vi "Test2_3a_ruben.vi"(7 "Report Enable":bool=TRUE, 8 "error in":errorcluster, 9 "Cycles Burst":i32=10000, 11 "Instrument VISA in":T1={"AWG VISA"="81160A", "Oscilloscope  VISA "="DSO80204B", "Integration Board IP"="172.16.7.43", "connection ID"=refnum, "report out"=refnum, "report file path"=path "D:/CTA/LevelTriggerBoardTest/TestsData/sumtrigger_delay/dataruben"}) -> (0 "error out":errorcluster, 3 "Instrument VISA out":T1={"AWG VISA"="81160A", "Oscilloscope  VISA "="DSO80204B", "Integration Board IP"="172.16.7.43", "connection ID"=refnum, "report out"=refnum, "report file path"=path "D:/CTA/LevelTriggerBoardTest/TestsData/sumtrigger_delay/dataruben"})   [LabVIEW 2009]
uses:
  <vilib>/Utility/NIReport.llb/NI_report.lvclass
  <vilib>/Utility/NIReport.llb/HTML/NI_HTML.lvclass
  <instrlib>/Agilent 8000 Series/Public/Configure/Configure Math (Binary Operation).vi
  <instrlib>/Agilent 81150/Agilent 81150.lvlib
  <instrlib>/Agilent 8000 Series/Agilent 8000 Series.lvlib
panel:
  in  "Quantity of measurements":u32
  in  "Delay Time (s)":dbl=10.0
  in  "Channel":i32=1
  in  "Points":i32=360
  in  "Save NOW!":bool
  in  "End 2":bool=TRUE
  out "Data output":dbl[][](array[numeric])=[[1.0, 1.0, 2200.0, 200.0, 0.0, 0.26, nan, 1.00955e-08, nan, 2.8861e-09, nan, 0.961, nan], [1.0, 1.0, 2200.0, 200.0, 1.0, 0.261, nan, 1.0146e-08, nan, 2.9059e-09, nan, 0.961, nan]]
  in  "sweep Vclip":T2={"MIN"=200.0, "MAX"=200.0, "Steps"=1.0, "Log scale"=FALSE}
  in  "sweep Vatt":T2={"MIN"=2200.0, "MAX"=2200.0, "Steps"=1.0, "Log scale"=FALSE}
  out "Measurement":dbl=0.261
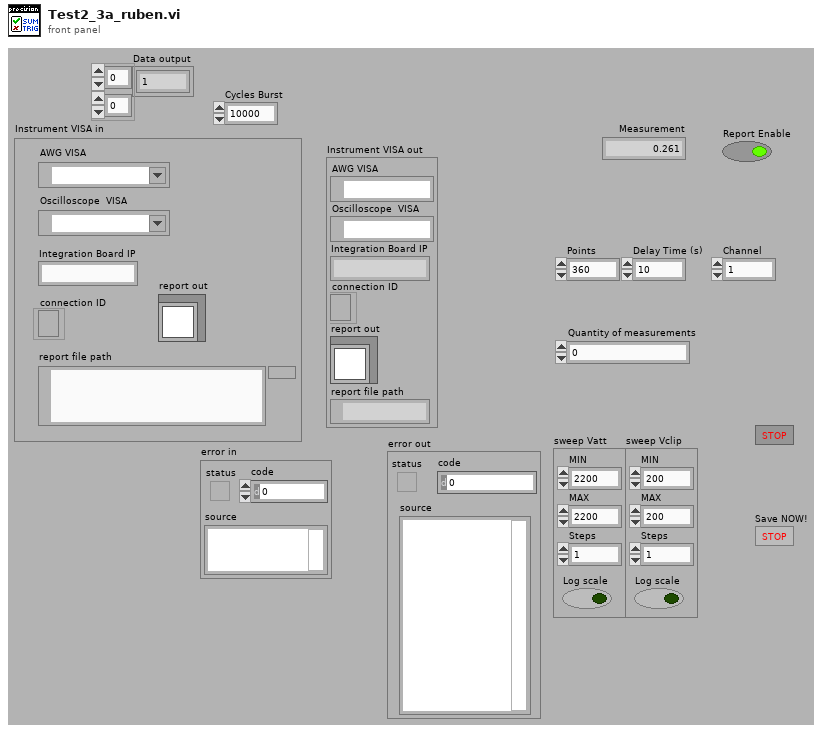
[diagram p1: front panel]
types:
  T1 = cluster{"AWG VISA":refnum<visa-resource-name>, "Oscilloscope  VISA ":refnum<visa-resource-name>, "Integration Board IP":string, "connection ID":refnum<k5>, "report out":refnum<class "NI_report.lvclass">, "report file path":path}
  T2 = cluster{"MIN":dbl, "MAX":dbl, "Steps":dbl, "Log scale":bool}
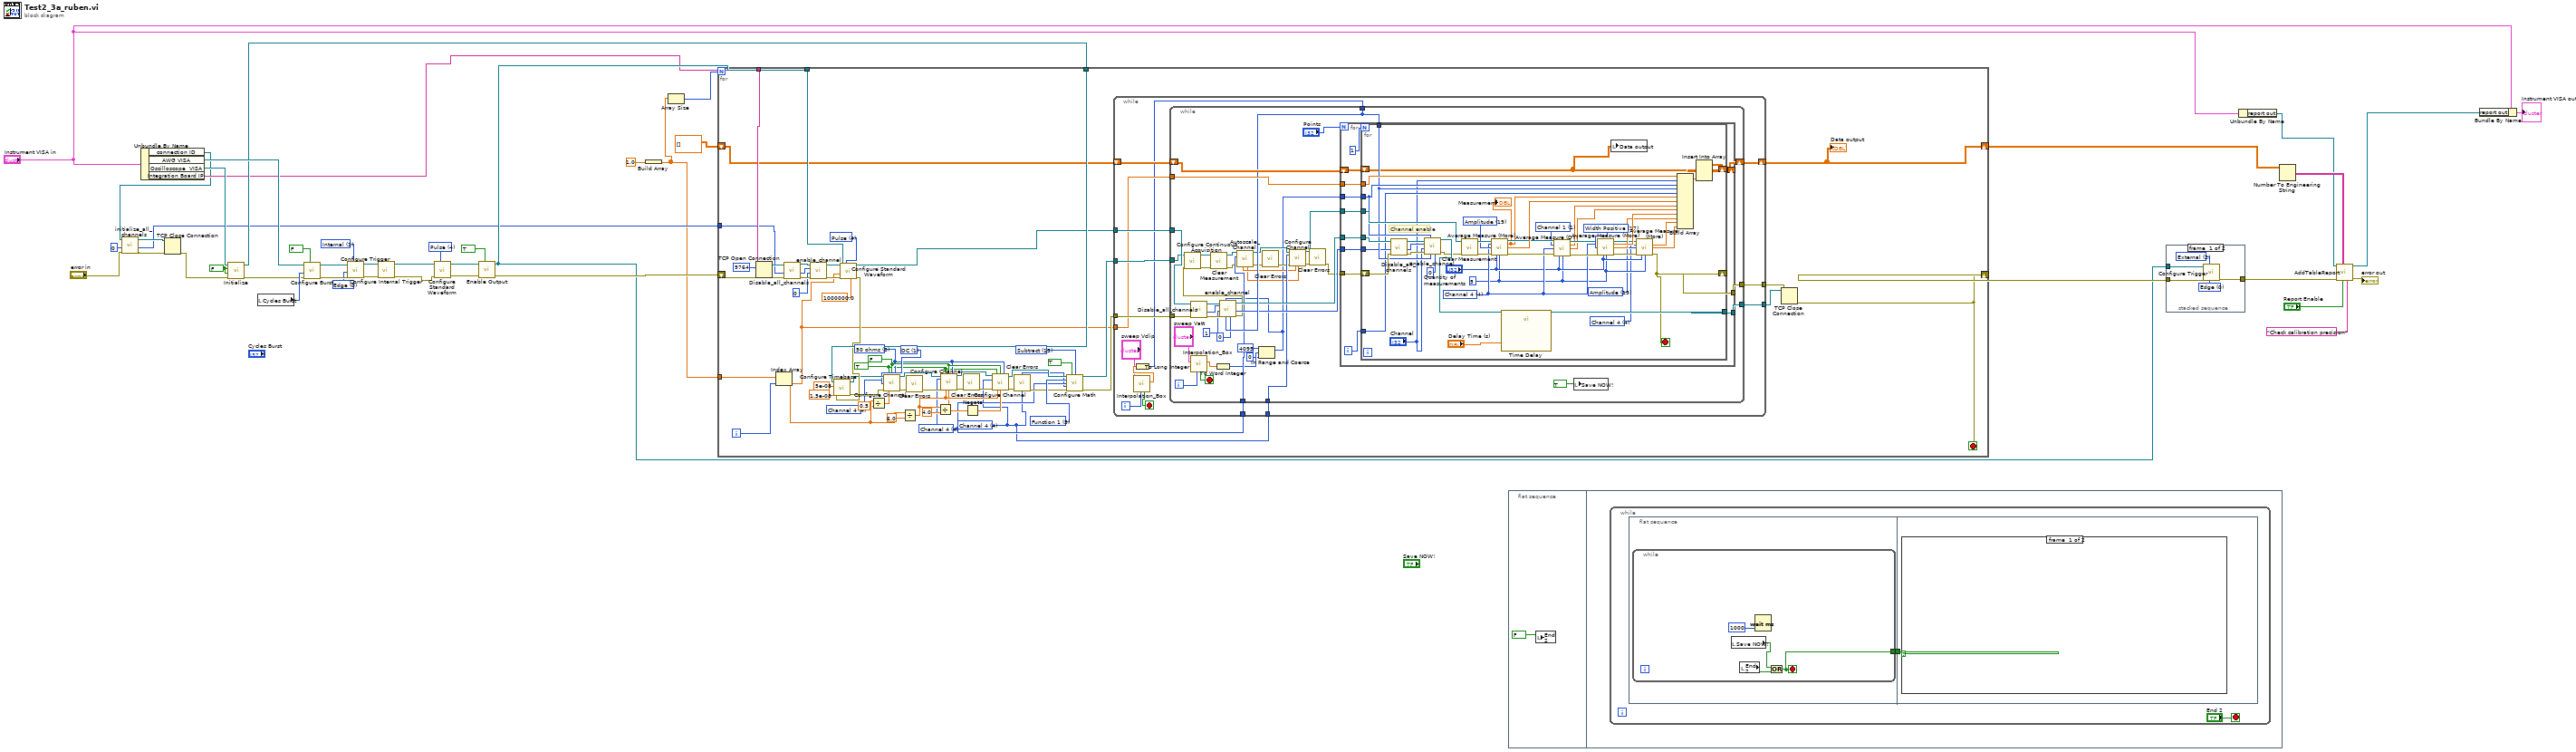
[diagram p0: block diagram]
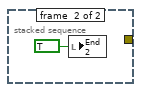
[diagram p2: hidden frame]
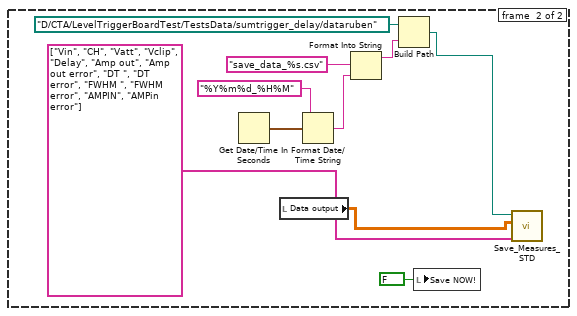
[diagram p3: hidden frame]
diagram:
  w26 = FALSE ("ID Query (True)")
  w33 = u16 1 items=["Immediate", "Internal", "External", "Software Trigger Function"] ("Trigger Source (0: Immediate)")
  w34 = u16 0 items=["Edge", "Level"] ("Trigger Mode (0: Edge)")
  w43 = u16 4 items=["Sine", "Square", "Ramp Up", "Ramp Down", "Pulse", "Noise", "DC"] ("Waveform (0: Sine)")
  n1 = Unbundle By Name("Instrument VISA in") -> ("connection ID"=w12:refnum<k5>, "AWG VISA"=w38:refnum<visa-resource-name>, "Oscilloscope  VISA"=w27:refnum<visa-resource-name>, "Integration Board IP"=w16:string)
  n2 = call "initialize_all_channels.vi"("error in"="error in", "id_in"=0, "connection ID"=w12) -> ("error out"=w14:errorcluster, "id_out"=w10:i32, "connection ID out"=w13:refnum<k5>)  [unwired: 6 in]
  n3 = TCP Close Connection(connection ID=w13, error in (no error)=w14) -> (error out=w19:errorcluster)  [unwired: 1 in, 1 out]
  n4 = call <instrlib>:"Initialize.vi"("error in (no error)"=w19, "Reset (True)"=w26, "ID Query (True)"=w26, "VISA resource name"=w27) -> ("error out"=w28:errorcluster, "VISA resource name out"=w17:refnum<visa-resource-name>)  [unwired: 6 in]
  n5 = local read "Cycles Burst"() -> (w39:i32)
  n6 = call <instrlib>:"Configure Burst.vi"("Enable Burst (F: Disable)"=FALSE, "error in (no error)"=w28, "Burst Count (2)"=w39, "VISA resource name"=w38) -> ("error out"=w36:errorcluster, "VISA resource name out"=w35:refnum<visa-resource-name>)  [unwired: 6 in]
  n7 = call <instrlib>:"Configure Trigger.vi"("Trigger Source (0: Immediate)"=w33, "error in (no error)"=w36, "Trigger Mode (0: Edge)"=w34, "VISA resource name"=w35) -> ("error out"=w32:errorcluster, "VISA resource name out"=w31:refnum<visa-resource-name>)  [unwired: 6 in]
  n8 = call <instrlib>:"Configure Internal Trigger.vi"("error in (no error)"=w32, "VISA resource name"=w31) -> ("error out"=w29:errorcluster, "VISA resource name out"=w30:refnum<visa-resource-name>)  [unwired: 8 in]
  n9 = call <instrlib>:"Configure Standard Waveform.vi"("Waveform (0: Sine)"=w43, "error in (no error)"=w29, "VISA resource name"=w30) -> ("error out"=w42:errorcluster, "VISA resource name out"=w41:refnum<visa-resource-name>)  [unwired: 7 in]
  n10 = call <instrlib>:"Enable Output.vi"("Enable Output (T: Enable)"=TRUE, "error in (no error)"=w42, "VISA resource name"=w41) -> ("error out"=w37:errorcluster, "VISA resource name out"=w18:refnum<visa-resource-name>)  [unwired: 7 in]
  n11 = Build Array(1.0 ("element")) -> (w2:dbl[])
  n12 = Array Size(array=w2) -> (size(s)=w1:i32)
  n13 = for {
    N: w1 -> [_]
    shift-right: [w93] -> w25
    shift-left: w37 -> [w96]
    tunnel: w18 -> [w99]
    tunnel: w17 -> [w90]
    tunnel: w16 -> [w95]
    tunnel: w10 -> [w63]
    shift-right: [w49] -> w9
    shift-left: dbl[][] [] -> [w52]
    tunnel: w2 -> [w48]
    i -> [w98]
    stop <- w93 stop-if-true
    w67 = TRUE ("Enable Channel (Enable)")
    w69 = FALSE ("BW Limit 20MHz (Disable)")
    w68 = u32 0 items=["50 ohms", "1 Mohms"] ("Input Impedance (1: 1 Mohms)")
    w79 = 4 items=["Channel 1"=1, "Channel 2"=2, "Channel 3"=3, "Channel 4"=4] ("Channel (1: Channel 1)")
    w80 = 1 items=["AC", "DC"] ("Vertical Coupling (1: DC)")
    w84 = u16 5 items=["Function 1"=5, "Function 2"=6, "Function 3"=7, "Function 4"=8] ("Math Channel (5: Function 1)")
    w85 = u16 15 items=["Add"=12, "Divide"=13, "Multiply"=14, "Subtract"=15, "Common Mode"=16, "Versus"=17] ("Math Operation (12: Add)")
    w51 = 4 items=["Channel 1"=1, "Channel 2"=2, "Channel 3"=3, "Channel 4"=4] ("Channel (1: Channel 1)")
    w50 = 4 items=["Channel 1"=1, "Channel 2"=2, "Channel 3"=3, "Channel 4"=4] ("Channel (1: Channel 1)")
    w100 = u16 4 items=["Sine", "Square", "Ramp Up", "Ramp Down", "Pulse", "Noise", "DC"] ("Waveform (0: Sine)")
    n14 = TCP Open Connection(address=w95, remote port or service name=u16 9764, error in (no error)=w96) -> (connection ID=w64:refnum<k5>, error out=w65:errorcluster)  [unwired: 2 in]
    n15 = Index Array(array=w48, index=w98) -> (element=w47:dbl)
    n16 = call "Disable_all_channels.vi"("error in"=w65, "id_in"=w63, "connection ID"=w64) -> ("error out"=w59:errorcluster, "id_out"=w58:i32, "connection ID out"=w61:refnum<k5>)  [unwired: 6 in]
    n17 = call "enable_channel.vi"("error in"=w59, "Channel"=u16 0 ("remote port or service name"), "id_in"=w58, "connection ID"=w61) -> ("error out"=w60:errorcluster, "connection ID out"=w62:refnum<k5>)  [unwired: 5 in, 1 out]
    n18 = call <instrlib>:"Configure Standard Waveform.vi"("Frequency (1000.0 Hz)"=1000000.0, "Waveform (0: Sine)"=w100, "error in (no error)"=w60, "Amplitude (1.0 Vpp)"=w47, "VISA resource name"=w99) -> ("error out"=w89:errorcluster)  [unwired: 5 in, 1 out]
    n19 = call <instrlib>:"Configure Timebase.vi"("error in (no error)"=w89, "Position (0.0 s)"=1.5e-08, "Timebase (0.005 s)"=5e-08, "VISA resource name"=w90) -> ("error out"=w81:errorcluster, "VISA resource name out"=w82:refnum<visa-resource-name>)  [unwired: 6 in]
    n20 = Divide(x=w47, y=0.5) -> (x/y=w45:dbl)
    n21 = call <instrlib>:"Configure Channel.vi"("VISA resource name"=w82, "Enable Channel (Enable)"=w67, "BW Limit 20MHz (Disable)"=w69, "Input Impedance (1: 1 Mohms)"=w68, "Channel (1: Channel 1)"=w79, "Vertical Coupling (1: DC)"=w80, "error in (no error)"=w81, "Vertical Range (2.0 V)"=w45) -> ("VISA resource name out"=w77:refnum<visa-resource-name>, "error out"=w78:errorcluster)  [unwired: 6 in]
    n22 = Divide(x=w47, y=6.0) -> (x/y=w56:dbl)
    n23 = call <vilib>:"Clear Errors.vi"("error in (no error)"=w78) -> ("error out"=w74:errorcluster)  [unwired: 6 in]
    n24 = Divide(x=w56, y=4.0) -> (x/y=w53:dbl)
    n25 = call <instrlib>:"Configure Channel.vi"("VISA resource name"=w77, "Enable Channel (Enable)"=w67, "BW Limit 20MHz (Disable)"=w69, "Input Impedance (1: 1 Mohms)"=w68, "Channel (1: Channel 1)"=w51, "error in (no error)"=w74, "Vertical Range (2.0 V)"=w56, "Vertical Offset (0.0 V)"=w53) -> ("VISA resource name out"=w76:refnum<visa-resource-name>, "error out"=w73:errorcluster)  [unwired: 6 in]
    n26 = call <vilib>:"Clear Errors.vi"("error in (no error)"=w73) -> ("error out"=w72:errorcluster)  [unwired: 6 in]
    n27 = Negate(x=w53) -> (-x=w54:dbl)
    n28 = call <instrlib>:"Configure Channel.vi"("VISA resource name"=w76, "Enable Channel (Enable)"=w67, "BW Limit 20MHz (Disable)"=w69, "Input Impedance (1: 1 Mohms)"=w68, "Channel (1: Channel 1)"=w50, "error in (no error)"=w72, "Vertical Range (2.0 V)"=w56, "Vertical Offset (0.0 V)"=w54) -> ("VISA resource name out"=w75:refnum<visa-resource-name>, "error out"=w71:errorcluster)  [unwired: 6 in]
    n29 = call <vilib>:"Clear Errors.vi"("error in (no error)"=w71) -> ("error out"=w70:errorcluster)  [unwired: 6 in]
    n30 = call-poly <instrlib>:"Configure Math.vi"("VISA resource name"=w75, "Enable Math Channel (T:Enable)"=TRUE, "Math Operation (12: Add)"=w85, "Math Channel (5: Function 1)"=w84, "Math Operand (1: Channel 1)"=w51, "Math Operand (2: Channel 2)"=w50, "error in (no error)"=w70) -> ("VISA resource name out"=w88:refnum<visa-resource-name>, "error out"=w87:errorcluster)  [unwired: 7 in]
    n31 = while {
      tunnel: [w116] -> w94
      tunnel: [w115] -> w92
      tunnel: w88 -> [w114]
      tunnel: w87 -> [w113]
      tunnel: w62 -> [w112]
      tunnel: w47 -> [w111]
      shift-right: [w110] -> w49
      shift-left: w52 -> [w109]
      tunnel: w51 -> [w108]
      tunnel: w50 -> [w107]
      i -> [w105]
      stop <- w106 stop-if-true
      n32 = call "Interpolation_Box.vi"("Current step"=w105, "sweep parameters"="sweep Vclip") -> ("Value"=w103:dbl, "Finished"=w106:bool)  [unwired: 7 in, 1 out]
      n33 = To Long Integer(number=w103) -> (32bit integer=w104:i32)
      n34 = while {
        tunnel: [w157] -> w116
        tunnel: [w156] -> w115
        tunnel: w114 -> [w127]
        tunnel: w113 -> [w151]
        tunnel: w112 -> [w148]
        tunnel: w111 -> [w155]
        shift-right: [w154] -> w110
        shift-left: w109 -> [w153]
        tunnel: w104 -> [w150]
        tunnel: w108 -> [w143]
        tunnel: w107 -> [w138]
        i -> [w132]
        stop <- w142 stop-if-true
        n35 = call "Interpolation_Box.vi"("Current step"=w132, "sweep parameters"="sweep Vatt") -> ("Value"=w131:dbl, "Finished"=w142:bool)  [unwired: 7 in, 1 out]
        n36 = call "Disable_all_channels.vi"("error in"=w151, "connection ID"=w148) -> ("error out"=w152:errorcluster, "id_out"=w146:i32, "connection ID out"=w149:refnum<k5>)  [unwired: 7 in]
        n37 = To Word Integer(number=w131) -> (16bit integer=w122:i16)
        n38 = In Range and Coerce(upper limit=i16 4095, x=w122, lower limit=i16 0) -> (coerced(x)=w119:i16)  [unwired: 1 out]
        n39 = call "enable_channel.vi"("Delay"=0, "V clip"=w150, "V att"=w119, "error in"=w152, "Channel"=u32 1 ("Max Errors"), "id_in"=w146, "connection ID"=w149) -> ("error out"=w125:errorcluster, "id_out"=w144:i32, "connection ID out"=w147:refnum<k5>)  [unwired: 2 in]
        n40 = call <instrlib>:"Configure Continuous Acquisition.vi"("error in (no error)"=w125, "VISA resource name"=w127) -> ("error out"=w124:errorcluster, "VISA resource name out"=w126:refnum<visa-resource-name>)  [unwired: 8 in]
        n41 = call <instrlib>:"Clear Measurement.vi"("error in (no error)"=w124, "VISA resource name"=w126) -> ("error out"=w129:errorcluster, "VISA resource name out"=w128:refnum<visa-resource-name>)  [unwired: 8 in]
        n42 = call "Autoscale_Channel.vi"("error in"=w129, "Channel"=w143, "VISA resource name"=w128) -> ("error out"=w133:errorcluster, "VISA resource name out"=w139:refnum<visa-resource-name>, "Offset"=w117:dbl, "VerticalRange"=w137:dbl)  [unwired: 5 in]
        n43 = call <vilib>:"Clear Errors.vi"("error in (no error)"=w133) -> ("error out"=w134:errorcluster)  [unwired: 6 in]
        n44 = call <instrlib>:"Configure Channel.vi"("VISA resource name"=w139, "Channel (1: Channel 1)"=w138, "error in (no error)"=w134, "Vertical Range (2.0 V)"=w137, "Vertical Offset (0.0 V)"=w117) -> ("VISA resource name out"=w140:refnum<visa-resource-name>, "error out"=w135:errorcluster)  [unwired: 9 in]
        n45 = call <vilib>:"Clear Errors.vi"("error in (no error)"=w135) -> ("error out"=w136:errorcluster)  [unwired: 6 in]
        n46 = for {
          N: "Points" -> [_]
          tunnel: [w169] -> w157
          tunnel: [w168] -> w156
          tunnel: w155 -> [w167]
          tunnel: w150 -> [w164]
          tunnel: w147 -> [w163]
          tunnel: w144 -> [w162]
          tunnel: w140 -> [w161]
          tunnel: w136 -> [w160]
          tunnel: w119 -> [w159]
          shift-right: [w166] -> w154
          shift-left: w153 -> [w165]
          i -> [w158]
          n47 = for {
            N: 1 -> [_]
            shift-right: [w178] -> w169
            shift-left: w160 -> [w211]
            tunnel: w163 -> [w212]
            tunnel: w161 -> [w208]
            tunnel: [w214] -> w168
            tunnel: w167 -> [w207]
            shift-right: [w205] -> w166
            shift-left: w165 -> [w183]
            tunnel: w159 -> [w187]
            tunnel: w164 -> [w186]
            tunnel: w162 -> [w185]
            tunnel: w158 -> [w184]
            stop <- w178 stop-if-true
            w174 = 4 items=["Channel 1"=1, "Channel 2"=2, "Channel 3"=3, "Channel 4"=4, "Function 1"=5, "Function 2"=6, "Function 3"=7, "Function 4"=8, "Memory 1"=9, "Memory 2"=10, "Memory 3"=11, "Memory 4"=12] ("Channel (1: Channel 1)")
            w175 = 19 items=["Rise Time", "Fall Time", "Frequency", "Period", "Voltage RMS(AC)", "Voltage RMS(DC)", "Voltage RMS (AC,cycle)", "Voltage RMS (DC,cycle)", "Voltage Max", "Voltage Min", "Voltage Middle", "Voltage Vpp", "Voltage High", "Voltage Low", "Voltage Average", "Voltage Average (cycle)", "Width Negative", "Width Positive", "Duty Cycle Positive", "Amplitude", "Overshoot", "Preshoot", "Voltage Base", "Voltage Upper", "Time Max", "Time Min", "Color Grade Crossing", "Color Grade Eye Width", "Color Grade Eye Height", "Color Grade Eye Q-Factory", "Color Grade Eye Duty Cycle Distortion(Percent)", "Color Grade Eye Duty Cycle Distortion(Time)", "Color Grade Eye Jitter(PP)", "Color Grade Eye Width(RMS)", "Cycle-cycle Duty Jitter(Rising)", "Cycle-cycle Duty Jitter(Falling)", "Cycle-cycle Jitter(Rising)", "Cycle-cycle Jitter(Falling)", "Cycle-cycle - Width", "Cycle-cycle + Width", "Date Rate", "Unit Interval", "FFT Delta Frequency", "FFT Delta Magnitude", "FFT Frequency", "FFT Magnitude", "Slew Rate", "Area (Entire Display)", "Area(Single Cycle)", "Duty Cycle (Rising)", "Duty Cycle (Falling)"] ("Measurement Function (0: Rise Time)")
            w176 = u32 5 ("Max Errors")
            w200 = 17 items=["Rise Time", "Fall Time", "Frequency", "Period", "Voltage RMS(AC)", "Voltage RMS(DC)", "Voltage RMS (AC,cycle)", "Voltage RMS (DC,cycle)", "Voltage Max", "Voltage Min", "Voltage Middle", "Voltage Vpp", "Voltage High", "Voltage Low", "Voltage Average", "Voltage Average (cycle)", "Width Negative", "Width Positive", "Duty Cycle Positive", "Amplitude", "Overshoot", "Preshoot", "Voltage Base", "Voltage Upper", "Time Max", "Time Min", "Color Grade Crossing", "Color Grade Eye Width", "Color Grade Eye Height", "Color Grade Eye Q-Factory", "Color Grade Eye Duty Cycle Distortion(Percent)", "Color Grade Eye Duty Cycle Distortion(Time)", "Color Grade Eye Jitter(PP)", "Color Grade Eye Width(RMS)", "Cycle-cycle Duty Jitter(Rising)", "Cycle-cycle Duty Jitter(Falling)", "Cycle-cycle Jitter(Rising)", "Cycle-cycle Jitter(Falling)", "Cycle-cycle - Width", "Cycle-cycle + Width", "Date Rate", "Unit Interval", "FFT Delta Frequency", "FFT Delta Magnitude", "FFT Frequency", "FFT Magnitude", "Slew Rate", "Area (Entire Display)", "Area(Single Cycle)", "Duty Cycle (Rising)", "Duty Cycle (Falling)"] ("Measurement Function (0: Rise Time)")
            w190 = u16 1 items=["Channel 1"=1, "Channel 2"=2, "Channel 3"=3, "Channel 4"=4, "Function 1"=5, "Function 2"=6, "Function 3"=7, "Function 4"=8, "Memory 1"=9, "Memory 2"=10, "Memory 3"=11, "Memory 4"=12] ("Channel1 (1: Channel 1)")
            w189 = 4 items=["Channel 1"=1, "Channel 2"=2, "Channel 3"=3, "Channel 4"=4, "Function 1"=5, "Function 2"=6, "Function 3"=7, "Function 4"=8, "Memory 1"=9, "Memory 2"=10, "Memory 3"=11, "Memory 4"=12] ("aa")
            w201 = 19 items=["Rise Time", "Fall Time", "Frequency", "Period", "Voltage RMS(AC)", "Voltage RMS(DC)", "Voltage RMS (AC,cycle)", "Voltage RMS (DC,cycle)", "Voltage Max", "Voltage Min", "Voltage Middle", "Voltage Vpp", "Voltage High", "Voltage Low", "Voltage Average", "Voltage Average (cycle)", "Width Negative", "Width Positive", "Duty Cycle Positive", "Amplitude", "Overshoot", "Preshoot", "Voltage Base", "Voltage Upper", "Time Max", "Time Min", "Color Grade Crossing", "Color Grade Eye Width", "Color Grade Eye Height", "Color Grade Eye Q-Factory", "Color Grade Eye Duty Cycle Distortion(Percent)", "Color Grade Eye Duty Cycle Distortion(Time)", "Color Grade Eye Jitter(PP)", "Color Grade Eye Width(RMS)", "Cycle-cycle Duty Jitter(Rising)", "Cycle-cycle Duty Jitter(Falling)", "Cycle-cycle Jitter(Rising)", "Cycle-cycle Jitter(Falling)", "Cycle-cycle - Width", "Cycle-cycle + Width", "Date Rate", "Unit Interval", "FFT Delta Frequency", "FFT Delta Magnitude", "FFT Frequency", "FFT Magnitude", "Slew Rate", "Area (Entire Display)", "Area(Single Cycle)", "Duty Cycle (Rising)", "Duty Cycle (Falling)"] ("Measurement Function (0: Rise Time)")
            # "Channel enable"
            n48 = call "Disable_all_channels.vi"("error in"=w211, "id_in"=w185, "connection ID"=w212) -> ("error out"=w210:errorcluster, "id_out"=w209:i32, "connection ID out"=w213:refnum<k5>)  [unwired: 6 in]
            n49 = call "enable_channel.vi"("Delay"=0, "V clip"=w186, "V att"=w187, "error in"=w210, "Channel"="Channel", "id_in"=w209, "connection ID"=w213) -> ("error out"=w188:errorcluster, "connection ID out"=w214:refnum<k5>)  [unwired: 2 in, 1 out]
            n50 = call <instrlib>:"Clear Measurement.vi"("error in (no error)"=w188, "VISA resource name"=w208) -> ("error out"=w202:errorcluster, "VISA resource name out"=w203:refnum<visa-resource-name>)  [unwired: 8 in]
            n51 = call "Average Measure (More).vi"("VISA resource name"=w203, "Channel (1: Channel 1)"=w189, "Measurement Function (0: Rise Time)"=w201, "error in (no error)"=w202, "Averages"="Quantity of measurements", "Max Errors"=w176) -> ("VISA resource name out"=w199:refnum<visa-resource-name>, "Measure Average"=w191:dbl, "Measure Error"=w204:dbl, "error out"=w196:errorcluster)  [unwired: 6 in]
            "Measurement" <- w191
            n52 = call "Time Delay"("Delay Time (s)"="Delay Time (s)") -> ()  [unwired: 10 in, 1 out]
            n53 = call "Average Measure (DT).vi"("VISA resource name"=w199, "Channel1 (1: Channel 1)"=w190, "Channel2 (2: Channel 2)"=w189, "error in (no error)"=w196, "Averages"="Quantity of measurements", "Max Errors"=w176) -> ("VISA resource name out"=w198:refnum<visa-resource-name>, "Measure Average"=w195:dbl, "Measure Error"=w194:dbl, "error out"=w197:errorcluster)  [unwired: 6 in]
            n54 = call "Average Measure (More).vi"("VISA resource name"=w198, "Channel (1: Channel 1)"=w189, "Measurement Function (0: Rise Time)"=w200, "error in (no error)"=w197, "Averages"="Quantity of measurements", "Max Errors"=w176) -> ("VISA resource name out"=w173:refnum<visa-resource-name>, "Measure Average"=w193:dbl, "Measure Error"=w192:dbl, "error out"=w179:errorcluster)  [unwired: 6 in]
            n55 = local write "Data output"(w183) -> ()
            n56 = call "Average Measure (More).vi"("VISA resource name"=w173, "Channel (1: Channel 1)"=w174, "Measurement Function (0: Rise Time)"=w175, "error in (no error)"=w179, "Averages"="Quantity of measurements", "Max Errors"=w176) -> ("Measure Average"=w172:dbl, "Measure Error"=w171:dbl, "error out"=w178:errorcluster)  [unwired: 6 in, 1 out]
            n57 = Build Array(w207, "Channel", w187, w186, w184, w191, w204, w195, w194, w193, w192, w172, w171) -> (w206:dbl[])
            n58 = Insert Into Array(array=w183, new element=w206) -> (w205:dbl[][])  [unwired: 2 in]
          }
        }
        n59 = local write "Save NOW!"(TRUE ("Save NOW! 2")) -> ()
      }
    }
    "Data output" <- w49
    n60 = TCP Close Connection(connection ID=w92, error in (no error)=w94) -> (error out=w93:errorcluster)  [unwired: 1 in, 1 out]
  }
  n61 = flat-sequence {
    frame #0 {
      n62 = local write "End 2"(FALSE ("End")) -> ()
    }
    frame #1 {
      n63 = while {
        stop <- "End 2" stop-if-true
        n64 = flat-sequence {
          tunnel: [w218] -> w216
          tunnel: w216 -> [w223]
          frame #0 {
            n65 = while {
              tunnel: [w219] -> w218
              stop <- w219 stop-if-true
              n66 = local read "Save NOW!"() -> (w220:bool)
              n67 = local read "End 2"() -> (w221:bool)
              n68 = Wait (ms)(milliseconds to wait=u32 1000) -> ()  [unwired: 1 out]
              n69 = Or(x=w220, y=w221) -> (x .or. y?=w219:bool)
            }
          }
          frame #1 {
            n70 = case shown="True" w223 {
              frame #0 {
              }
              frame #1 {
                n71 = Get Date/Time In Seconds() -> (seconds since 1Jan1904=w232:timestamp)
                n72 = local read "Data output"() -> (w225:dbl[][])
                n73 = Format Date/Time String(time format string (%c)="%Y%m%d_%H%M", seconds (now)=w232) -> (date/time string=w230:string)  [unwired: 1 in]
                n74 = Format Into String(format string="save_data_%s.csv", w230) -> (resulting string=w229:string)  [unwired: 2 in, 1 out]
                n75 = Build Path(base path=path "D:/CTA/LevelTriggerBoardTest/TestsData/sumtrigger_delay/dataruben", name or relative path=w229) -> (appended path=w228:path)
                n76 = local write "Save NOW!"(FALSE ("Save NOW!")) -> ()
                n77 = call "Save_Measures_STD.vi"("appended array"=string[] ["Vin", "CH", "Vatt", "Vclip", "Delay", "Amp out", "Amp out error", "DT ", "DT error", "FWHM ", "FWHM error", "AMPIN", "AMPin error"], "Data in"=w225, "file path (dialog if empty)"=w228) -> ()  [unwired: 9 in]
              }
            }
          }
        }
      }
    }
  }
  n78 = stacked-sequence {
    tunnel: w25 -> [w236 _]
    tunnel: [w235 _] -> w21
    tunnel: w18 -> [w234 _]
    frame #0 {
      w237 = u16 2 items=["Immediate", "Internal", "External", "Software Trigger Function"] ("Trigger Source (0: Immediate)")
      w238 = u16 0 items=["Edge", "Level"] ("Trigger Mode (0: Edge)")
      n79 = call <instrlib>:"Configure Trigger.vi"("Trigger Source (0: Immediate)"=w237, "error in (no error)"=w236, "Trigger Mode (0: Edge)"=w238, "VISA resource name"=w234) -> ("error out"=w235:errorcluster)  [unwired: 6 in, 1 out]
    }
    frame #1 {
      n80 = local write "End 2"(TRUE ("End 2")) -> ()
    }
  }
  n81 = Unbundle By Name("Instrument VISA in") -> ("report out"=w6:refnum<class "NI_report.lvclass">)
  n82 = Number To Engineering String(4:w9) -> (0:w7:string[][])  [unwired: 3 in]
  n83 = call "AddTableReport.vi"("Table title"="Check calibration precision", "Report Enable"="Report Enable", "Data"=w7, "error in"=w21, "report in"=w6) -> ("error out"=→"error out":errorcluster, "report out"=w22:refnum<class "NI_report.lvclass">)  [unwired: 5 in]
  n84 = Bundle By Name(cluster="Instrument VISA in", "report out"=w22) -> (→"Instrument VISA out":T1)
